vi "4.5 CSM API String to Numeric - Enum.vi"() -> ()   [LabVIEW 2017]
uses:
  <userlib>/_NEVSTOP/Communicable State Machine(CSM)/Communicable State Machine.lvlib
  API-String-Arugments-Support/API String Arguments Support.lvlib
panel:
  out "API String (I32 Channel)":T1(array[cluster])=[{"API String (I32 Channel)"="0", "Channel"=enum."CH1", "Channel"=enum."CH1"}, {"API String (I32 Channel)"="1", "Channel"=enum."CH1", "Channel"=enum."CH2"}, {"API String (I32 Channel)"="2", "Channel"=enum."CH1", "Channel"=enum."CH3"}, {"API String (I32 Channel)"="3", "Channel"=enum."CH1", "Channel"=enum."CH4"}, {"API String (I32 Channel)"="4", "Channel"=enum."CH1", "Channel"=enum."CH5"}, {"API String (I32 Channel)"="5", "Channel"=enum."CH1", "Channel"=enum."CH6"}, {"API String (I32 Channel)"="6", "Channel"=enum."CH1", "Channel"=enum."CH7"}, {"API String (I32 Channel)"="7", "Channel"=enum."CH1", "Channel"=enum."CH8"}, {"API String (I32 Channel)"="8", "Channel"=enum."CH1", "Channel"=enum."CH9"}, {"API String (I32 Channel)"="9", "Channel"=enum."CH1", "Channel"=enum."CH10"}, {"API String (I32 Channel)"="10", "Channel"=enum."CH1", "Channel"=enum."CH11"}, {"API String (I32 Channel)"="11", "Channel"=enum."CH1", "Channel"=enum."CH12"}, {"API String (I32 Channel)"="12", "Channel"=enum."CH1", "Channel"=enum."CH13"}, {"API String (I32 Channel)"="13", "Channel"=enum."CH1", "Channel"=enum."CH14"}, {"API String (I32 Channel)"="14", "Channel"=enum."CH1", "Channel"=enum."CH15"}, {"API String (I32 Channel)"="15", "Channel"=enum."CH1", "Channel"=enum."CH16"}]
  out "API String (Channel)":T2(array[cluster])=[{"API String (Channel)"="CH1", "Channel"=enum."CH1", "Channel"=enum."CH1"}, {"API String (Channel)"="CH2", "Channel"=enum."CH1", "Channel"=enum."CH2"}, {"API String (Channel)"="CH3", "Channel"=enum."CH1", "Channel"=enum."CH3"}, {"API String (Channel)"="CH4", "Channel"=enum."CH1", "Channel"=enum."CH4"}, {"API String (Channel)"="CH5", "Channel"=enum."CH1", "Channel"=enum."CH5"}, {"API String (Channel)"="CH6", "Channel"=enum."CH1", "Channel"=enum."CH6"}, {"API String (Channel)"="CH7", "Channel"=enum."CH1", "Channel"=enum."CH7"}, {"API String (Channel)"="CH8", "Channel"=enum."CH1", "Channel"=enum."CH8"}, {"API String (Channel)"="CH9", "Channel"=enum."CH1", "Channel"=enum."CH9"}, {"API String (Channel)"="CH10", "Channel"=enum."CH1", "Channel"=enum."CH10"}, {"API String (Channel)"="CH11", "Channel"=enum."CH1", "Channel"=enum."CH11"}, {"API String (Channel)"="CH12", "Channel"=enum."CH1", "Channel"=enum."CH12"}, {"API String (Channel)"="CH13", "Channel"=enum."CH1", "Channel"=enum."CH13"}, {"API String (Channel)"="CH14", "Channel"=enum."CH1", "Channel"=enum."CH14"}, {"API String (Channel)"="CH15", "Channel"=enum."CH1", "Channel"=enum."CH15"}, {"API String (Channel)"="CH16", "Channel"=enum."CH1", "Channel"=enum."CH16"}]
  out "API String (I32 Voltage)":T3(array[cluster])=[{"API String (I32 Voltage)"="0", "Enum (Vertical)"=enum."2mV", "Retrieved Vertical"=enum."1mV"}, {"API String (I32 Voltage)"="1", "Enum (Vertical)"=enum."2mV", "Retrieved Vertical"=enum."2mV"}, {"API String (I32 Voltage)"="2", "Enum (Vertical)"=enum."2mV", "Retrieved Vertical"=enum."5mV"}, {"API String (I32 Voltage)"="3", "Enum (Vertical)"=enum."2mV", "Retrieved Vertical"=enum."10mV"}, {"API String (I32 Voltage)"="4", "Enum (Vertical)"=enum."2mV", "Retrieved Vertical"=enum."20mV"}, {"API String (I32 Voltage)"="5", "Enum (Vertical)"=enum."2mV", "Retrieved Vertical"=enum."50mV"}, {"API String (I32 Voltage)"="6", "Enum (Vertical)"=enum."2mV", "Retrieved Vertical"=enum."100mV"}, {"API String (I32 Voltage)"="7", "Enum (Vertical)"=enum."2mV", "Retrieved Vertical"=enum."200mV"}, {"API String (I32 Voltage)"="8", "Enum (Vertical)"=enum."2mV", "Retrieved Vertical"=enum."500mV"}, {"API String (I32 Voltage)"="9", "Enum (Vertical)"=enum."2mV", "Retrieved Vertical"=enum."1V"}, {"API String (I32 Voltage)"="10", "Enum (Vertical)"=enum."2mV", "Retrieved Vertical"=enum."2V"}, {"API String (I32 Voltage)"="11", "Enum (Vertical)"=enum."2mV", "Retrieved Vertical"=enum."5V"}, {"API String (I32 Voltage)"="12", "Enum (Vertical)"=enum."2mV", "Retrieved Vertical"=enum."10V"}, {"API String (I32 Voltage)"="13", "Enum (Vertical)"=enum."2mV", "Retrieved Vertical"=enum."20V"}, {"API String (I32 Voltage)"="14", "Enum (Vertical)"=enum."2mV", "Retrieved Vertical"=enum."50V"}, {"API String (I32 Voltage)"="15", "Enum (Vertical)"=enum."2mV", "Retrieved Vertical"=enum."100V"}, {"API String (I32 Voltage)"="16", "Enum (Vertical)"=enum."2mV", "Retrieved Vertical"=enum."200V"}, {"API String (I32 Voltage)"="17", "Enum (Vertical)"=enum."2mV", "Retrieved Vertical"=enum."500V"}, {"API String (I32 Voltage)"="18", "Enum (Vertical)"=enum."2mV", "Retrieved Vertical"=enum."1kV"}, {"API String (I32 Voltage)"="19", "Enum (Vertical)"=enum."2mV", "Retrieved Vertical"=enum."2kV"}, {"API String (I32 Voltage)"="20", "Enum (Vertical)"=enum."2mV", "Retrieved Vertical"=enum."5kV"}, {"API String (I32 Voltage)"="21", "Enum (Vertical)"=enum."2mV", "Retrieved Vertical"=enum."10kV"}, {"API String (I32 Voltage)"="22", "Enum (Vertical)"=enum."2mV", "Retrieved Vertical"=enum."20kV"}]
  out "API String (SI Voltage)":T4(array[cluster])=[{"API String (SI Voltage)"="1mV", "Enum (Vertical)"=enum."2mV", "Retrieved Vertical"=enum."1mV"}, {"API String (SI Voltage)"="2mV", "Enum (Vertical)"=enum."2mV", "Retrieved Vertical"=enum."2mV"}, {"API String (SI Voltage)"="5mV", "Enum (Vertical)"=enum."2mV", "Retrieved Vertical"=enum."5mV"}, {"API String (SI Voltage)"="10mV", "Enum (Vertical)"=enum."2mV", "Retrieved Vertical"=enum."10mV"}, {"API String (SI Voltage)"="20mV", "Enum (Vertical)"=enum."2mV", "Retrieved Vertical"=enum."20mV"}, {"API String (SI Voltage)"="50mV", "Enum (Vertical)"=enum."2mV", "Retrieved Vertical"=enum."50mV"}, {"API String (SI Voltage)"="100mV", "Enum (Vertical)"=enum."2mV", "Retrieved Vertical"=enum."100mV"}, {"API String (SI Voltage)"="200mV", "Enum (Vertical)"=enum."2mV", "Retrieved Vertical"=enum."200mV"}, {"API String (SI Voltage)"="500mV", "Enum (Vertical)"=enum."2mV", "Retrieved Vertical"=enum."500mV"}, {"API String (SI Voltage)"="1V", "Enum (Vertical)"=enum."2mV", "Retrieved Vertical"=enum."1V"}, {"API String (SI Voltage)"="2V", "Enum (Vertical)"=enum."2mV", "Retrieved Vertical"=enum."2V"}, {"API String (SI Voltage)"="5V", "Enum (Vertical)"=enum."2mV", "Retrieved Vertical"=enum."5V"}, {"API String (SI Voltage)"="10V", "Enum (Vertical)"=enum."2mV", "Retrieved Vertical"=enum."10V"}, {"API String (SI Voltage)"="20V", "Enum (Vertical)"=enum."2mV", "Retrieved Vertical"=enum."20V"}, {"API String (SI Voltage)"="50V", "Enum (Vertical)"=enum."2mV", "Retrieved Vertical"=enum."50V"}, {"API String (SI Voltage)"="100V", "Enum (Vertical)"=enum."2mV", "Retrieved Vertical"=enum."100V"}, {"API String (SI Voltage)"="200V", "Enum (Vertical)"=enum."2mV", "Retrieved Vertical"=enum."200V"}, {"API String (SI Voltage)"="500V", "Enum (Vertical)"=enum."2mV", "Retrieved Vertical"=enum."500V"}, {"API String (SI Voltage)"="1kV", "Enum (Vertical)"=enum."2mV", "Retrieved Vertical"=enum."1kV"}, {"API String (SI Voltage)"="2kV", "Enum (Vertical)"=enum."2mV", "Retrieved Vertical"=enum."2kV"}, {"API String (SI Voltage)"="5kV", "Enum (Vertical)"=enum."2mV", "Retrieved Vertical"=enum."5kV"}, {"API String (SI Voltage)"="10kV", "Enum (Vertical)"=enum."2mV", "Retrieved Vertical"=enum."10kV"}, {"API String (SI Voltage)"="20kV", "Enum (Vertical)"=enum."2mV", "Retrieved Vertical"=enum."20kV"}]
  out "API String (I32 Time)":T5(array[cluster])=[{"API String (I32)"="0", "Enum (Time/Division)"=enum."1us", "Retrieved Enum"=enum."100ns"}, {"API String (I32)"="1", "Enum (Time/Division)"=enum."1us", "Retrieved Enum"=enum."200ns"}, {"API String (I32)"="2", "Enum (Time/Division)"=enum."1us", "Retrieved Enum"=enum."500ns"}, {"API String (I32)"="3", "Enum (Time/Division)"=enum."1us", "Retrieved Enum"=enum."1us"}, {"API String (I32)"="4", "Enum (Time/Division)"=enum."1us", "Retrieved Enum"=enum."2us"}, {"API String (I32)"="5", "Enum (Time/Division)"=enum."1us", "Retrieved Enum"=enum."5us"}, {"API String (I32)"="6", "Enum (Time/Division)"=enum."1us", "Retrieved Enum"=enum."10us"}, {"API String (I32)"="7", "Enum (Time/Division)"=enum."1us", "Retrieved Enum"=enum."20us"}, {"API String (I32)"="8", "Enum (Time/Division)"=enum."1us", "Retrieved Enum"=enum."50us"}, {"API String (I32)"="9", "Enum (Time/Division)"=enum."1us", "Retrieved Enum"=enum."100us"}, {"API String (I32)"="10", "Enum (Time/Division)"=enum."1us", "Retrieved Enum"=enum."200us"}, {"API String (I32)"="11", "Enum (Time/Division)"=enum."1us", "Retrieved Enum"=enum."500us"}, {"API String (I32)"="12", "Enum (Time/Division)"=enum."1us", "Retrieved Enum"=enum."1ms"}, {"API String (I32)"="13", "Enum (Time/Division)"=enum."1us", "Retrieved Enum"=enum."2ms"}, {"API String (I32)"="14", "Enum (Time/Division)"=enum."1us", "Retrieved Enum"=enum."5ms"}, {"API String (I32)"="15", "Enum (Time/Division)"=enum."1us", "Retrieved Enum"=enum."10ms"}, {"API String (I32)"="16", "Enum (Time/Division)"=enum."1us", "Retrieved Enum"=enum."20ms"}, {"API String (I32)"="17", "Enum (Time/Division)"=enum."1us", "Retrieved Enum"=enum."50ms"}, {"API String (I32)"="18", "Enum (Time/Division)"=enum."1us", "Retrieved Enum"=enum."100ms"}, {"API String (I32)"="19", "Enum (Time/Division)"=enum."1us", "Retrieved Enum"=enum."200ms"}, {"API String (I32)"="20", "Enum (Time/Division)"=enum."1us", "Retrieved Enum"=enum."500ms"}, {"API String (I32)"="21", "Enum (Time/Division)"=enum."1us", "Retrieved Enum"=enum."1s"}, {"API String (I32)"="22", "Enum (Time/Division)"=enum."1us", "Retrieved Enum"=enum."2s"}, {"API String (I32)"="23", "Enum (Time/Division)"=enum."1us", "Retrieved Enum"=enum."3s"}, {"API String (I32)"="24", "Enum (Time/Division)"=enum."1us", "Retrieved Enum"=enum."4s"}, {"API String (I32)"="25", "Enum (Time/Division)"=enum."1us", "Retrieved Enum"=enum."5s"}, {"API String (I32)"="26", "Enum (Time/Division)"=enum."1us", "Retrieved Enum"=enum."6s"}, {"API String (I32)"="27", "Enum (Time/Division)"=enum."1us", "Retrieved Enum"=enum."8s"}, {"API String (I32)"="28", "Enum (Time/Division)"=enum."1us", "Retrieved Enum"=enum."10s"}, {"API String (I32)"="29", "Enum (Time/Division)"=enum."1us", "Retrieved Enum"=enum."20s"}, {"API String (I32)"="30", "Enum (Time/Division)"=enum."1us", "Retrieved Enum"=enum."30s"}, {"API String (I32)"="31", "Enum (Time/Division)"=enum."1us", "Retrieved Enum"=enum."1min"}, {"API String (I32)"="32", "Enum (Time/Division)"=enum."1us", "Retrieved Enum"=enum."2min"}, {"API String (I32)"="33", "Enum (Time/Division)"=enum."1us", "Retrieved Enum"=enum."3min"}, {"API String (I32)"="34", "Enum (Time/Division)"=enum."1us", "Retrieved Enum"=enum."4min"}, {"API String (I32)"="35", "Enum (Time/Division)"=enum."1us", "Retrieved Enum"=enum."5min"}, {"API String (I32)"="36", "Enum (Time/Division)"=enum."1us", "Retrieved Enum"=enum."6min"}, {"API String (I32)"="37", "Enum (Time/Division)"=enum."1us", "Retrieved Enum"=enum."7min"}, {"API String (I32)"="38", "Enum (Time/Division)"=enum."1us", "Retrieved Enum"=enum."8min"}, {"API String (I32)"="39", "Enum (Time/Division)"=enum."1us", "Retrieved Enum"=enum."9min"}, {"API String (I32)"="40", "Enum (Time/Division)"=enum."1us", "Retrieved Enum"=enum."10min"}, {"API String (I32)"="41", "Enum (Time/Division)"=enum."1us", "Retrieved Enum"=enum."12min"}, {"API String (I32)"="42", "Enum (Time/Division)"=enum."1us", "Retrieved Enum"=enum."15min"}, {"API String (I32)"="43", "Enum (Time/Division)"=enum."1us", "Retrieved Enum"=enum."30min"}, {"API String (I32)"="44", "Enum (Time/Division)"=enum."1us", "Retrieved Enum"=enum."1hour"}, {"API String (I32)"="45", "Enum (Time/Division)"=enum."1us", "Retrieved Enum"=enum."2hour"}, {"API String (I32)"="46", "Enum (Time/Division)"=enum."1us", "Retrieved Enum"=enum."3hour"}, {"API String (I32)"="47", "Enum (Time/Division)"=enum."1us", "Retrieved Enum"=enum."4hour"}, {"API String (I32)"="48", "Enum (Time/Division)"=enum."1us", "Retrieved Enum"=enum."5hour"}, {"API String (I32)"="49", "Enum (Time/Division)"=enum."1us", "Retrieved Enum"=enum."6hour"}, {"API String (I32)"="50", "Enum (Time/Division)"=enum."1us", "Retrieved Enum"=enum."7hour"}, {"API String (I32)"="51", "Enum (Time/Division)"=enum."1us", "Retrieved Enum"=enum."8hour"}, {"API String (I32)"="52", "Enum (Time/Division)"=enum."1us", "Retrieved Enum"=enum."9hour"}, {"API String (I32)"="53", "Enum (Time/Division)"=enum."1us", "Retrieved Enum"=enum."10hour"}, {"API String (I32)"="54", "Enum (Time/Division)"=enum."1us", "Retrieved Enum"=enum."12hour"}, {"API String (I32)"="55", "Enum (Time/Division)"=enum."1us", "Retrieved Enum"=enum."1day"}, {"API String (I32)"="56", "Enum (Time/Division)"=enum."1us", "Retrieved Enum"=enum."2day"}, {"API String (I32)"="57", "Enum (Time/Division)"=enum."1us", "Retrieved Enum"=enum."3day"}]
  out "API String (SI Time)":T6(array[cluster])=[{"API String (SI Format)"="100ns", "Enum (Time/Division)"=enum."1us", "Retrieved Enum"=enum."100ns"}, {"API String (SI Format)"="200ns", "Enum (Time/Division)"=enum."1us", "Retrieved Enum"=enum."200ns"}, {"API String (SI Format)"="500ns", "Enum (Time/Division)"=enum."1us", "Retrieved Enum"=enum."500ns"}, {"API String (SI Format)"="1us", "Enum (Time/Division)"=enum."1us", "Retrieved Enum"=enum."1us"}, {"API String (SI Format)"="2us", "Enum (Time/Division)"=enum."1us", "Retrieved Enum"=enum."2us"}, {"API String (SI Format)"="5us", "Enum (Time/Division)"=enum."1us", "Retrieved Enum"=enum."5us"}, {"API String (SI Format)"="10us", "Enum (Time/Division)"=enum."1us", "Retrieved Enum"=enum."10us"}, {"API String (SI Format)"="20us", "Enum (Time/Division)"=enum."1us", "Retrieved Enum"=enum."20us"}, {"API String (SI Format)"="50us", "Enum (Time/Division)"=enum."1us", "Retrieved Enum"=enum."50us"}, {"API String (SI Format)"="100us", "Enum (Time/Division)"=enum."1us", "Retrieved Enum"=enum."100us"}, {"API String (SI Format)"="200us", "Enum (Time/Division)"=enum."1us", "Retrieved Enum"=enum."200us"}, {"API String (SI Format)"="500us", "Enum (Time/Division)"=enum."1us", "Retrieved Enum"=enum."500us"}, {"API String (SI Format)"="1ms", "Enum (Time/Division)"=enum."1us", "Retrieved Enum"=enum."1ms"}, {"API String (SI Format)"="2ms", "Enum (Time/Division)"=enum."1us", "Retrieved Enum"=enum."2ms"}, {"API String (SI Format)"="5ms", "Enum (Time/Division)"=enum."1us", "Retrieved Enum"=enum."5ms"}, {"API String (SI Format)"="10ms", "Enum (Time/Division)"=enum."1us", "Retrieved Enum"=enum."10ms"}, {"API String (SI Format)"="20ms", "Enum (Time/Division)"=enum."1us", "Retrieved Enum"=enum."20ms"}, {"API String (SI Format)"="50ms", "Enum (Time/Division)"=enum."1us", "Retrieved Enum"=enum."50ms"}, {"API String (SI Format)"="100ms", "Enum (Time/Division)"=enum."1us", "Retrieved Enum"=enum."100ms"}, {"API String (SI Format)"="200ms", "Enum (Time/Division)"=enum."1us", "Retrieved Enum"=enum."200ms"}, {"API String (SI Format)"="500ms", "Enum (Time/Division)"=enum."1us", "Retrieved Enum"=enum."500ms"}, {"API String (SI Format)"="1s", "Enum (Time/Division)"=enum."1us", "Retrieved Enum"=enum."1s"}, {"API String (SI Format)"="2s", "Enum (Time/Division)"=enum."1us", "Retrieved Enum"=enum."2s"}, {"API String (SI Format)"="3s", "Enum (Time/Division)"=enum."1us", "Retrieved Enum"=enum."3s"}, {"API String (SI Format)"="4s", "Enum (Time/Division)"=enum."1us", "Retrieved Enum"=enum."4s"}, {"API String (SI Format)"="5s", "Enum (Time/Division)"=enum."1us", "Retrieved Enum"=enum."5s"}, {"API String (SI Format)"="6s", "Enum (Time/Division)"=enum."1us", "Retrieved Enum"=enum."6s"}, {"API String (SI Format)"="8s", "Enum (Time/Division)"=enum."1us", "Retrieved Enum"=enum."8s"}, {"API String (SI Format)"="10s", "Enum (Time/Division)"=enum."1us", "Retrieved Enum"=enum."10s"}, {"API String (SI Format)"="20s", "Enum (Time/Division)"=enum."1us", "Retrieved Enum"=enum."20s"}, {"API String (SI Format)"="30s", "Enum (Time/Division)"=enum."1us", "Retrieved Enum"=enum."30s"}, {"API String (SI Format)"="1min", "Enum (Time/Division)"=enum."1us", "Retrieved Enum"=enum."1min"}, {"API String (SI Format)"="2min", "Enum (Time/Division)"=enum."1us", "Retrieved Enum"=enum."2min"}, {"API String (SI Format)"="3min", "Enum (Time/Division)"=enum."1us", "Retrieved Enum"=enum."3min"}, {"API String (SI Format)"="4min", "Enum (Time/Division)"=enum."1us", "Retrieved Enum"=enum."4min"}, {"API String (SI Format)"="5min", "Enum (Time/Division)"=enum."1us", "Retrieved Enum"=enum."5min"}, {"API String (SI Format)"="6min", "Enum (Time/Division)"=enum."1us", "Retrieved Enum"=enum."6min"}, {"API String (SI Format)"="7min", "Enum (Time/Division)"=enum."1us", "Retrieved Enum"=enum."7min"}, {"API String (SI Format)"="8min", "Enum (Time/Division)"=enum."1us", "Retrieved Enum"=enum."8min"}, {"API String (SI Format)"="9min", "Enum (Time/Division)"=enum."1us", "Retrieved Enum"=enum."9min"}, {"API String (SI Format)"="10min", "Enum (Time/Division)"=enum."1us", "Retrieved Enum"=enum."10min"}, {"API String (SI Format)"="12min", "Enum (Time/Division)"=enum."1us", "Retrieved Enum"=enum."12min"}, {"API String (SI Format)"="15min", "Enum (Time/Division)"=enum."1us", "Retrieved Enum"=enum."15min"}, {"API String (SI Format)"="30min", "Enum (Time/Division)"=enum."1us", "Retrieved Enum"=enum."30min"}, {"API String (SI Format)"="1hour", "Enum (Time/Division)"=enum."1us", "Retrieved Enum"=enum."1hour"}, {"API String (SI Format)"="2hour", "Enum (Time/Division)"=enum."1us", "Retrieved Enum"=enum."2hour"}, {"API String (SI Format)"="3hour", "Enum (Time/Division)"=enum."1us", "Retrieved Enum"=enum."3hour"}, {"API String (SI Format)"="4hour", "Enum (Time/Division)"=enum."1us", "Retrieved Enum"=enum."4hour"}, {"API String (SI Format)"="5hour", "Enum (Time/Division)"=enum."1us", "Retrieved Enum"=enum."5hour"}, {"API String (SI Format)"="6hour", "Enum (Time/Division)"=enum."1us", "Retrieved Enum"=enum."6hour"}, {"API String (SI Format)"="7hour", "Enum (Time/Division)"=enum."1us", "Retrieved Enum"=enum."7hour"}, {"API String (SI Format)"="8hour", "Enum (Time/Division)"=enum."1us", "Retrieved Enum"=enum."8hour"}, {"API String (SI Format)"="9hour", "Enum (Time/Division)"=enum."1us", "Retrieved Enum"=enum."9hour"}, {"API String (SI Format)"="10hour", "Enum (Time/Division)"=enum."1us", "Retrieved Enum"=enum."10hour"}, {"API String (SI Format)"="12hour", "Enum (Time/Division)"=enum."1us", "Retrieved Enum"=enum."12hour"}, {"API String (SI Format)"="1day", "Enum (Time/Division)"=enum."1us", "Retrieved Enum"=enum."1day"}, {"API String (SI Format)"="2day", "Enum (Time/Division)"=enum."1us", "Retrieved Enum"=enum."2day"}, {"API String (SI Format)"="3day", "Enum (Time/Division)"=enum."1us", "Retrieved Enum"=enum."3day"}]
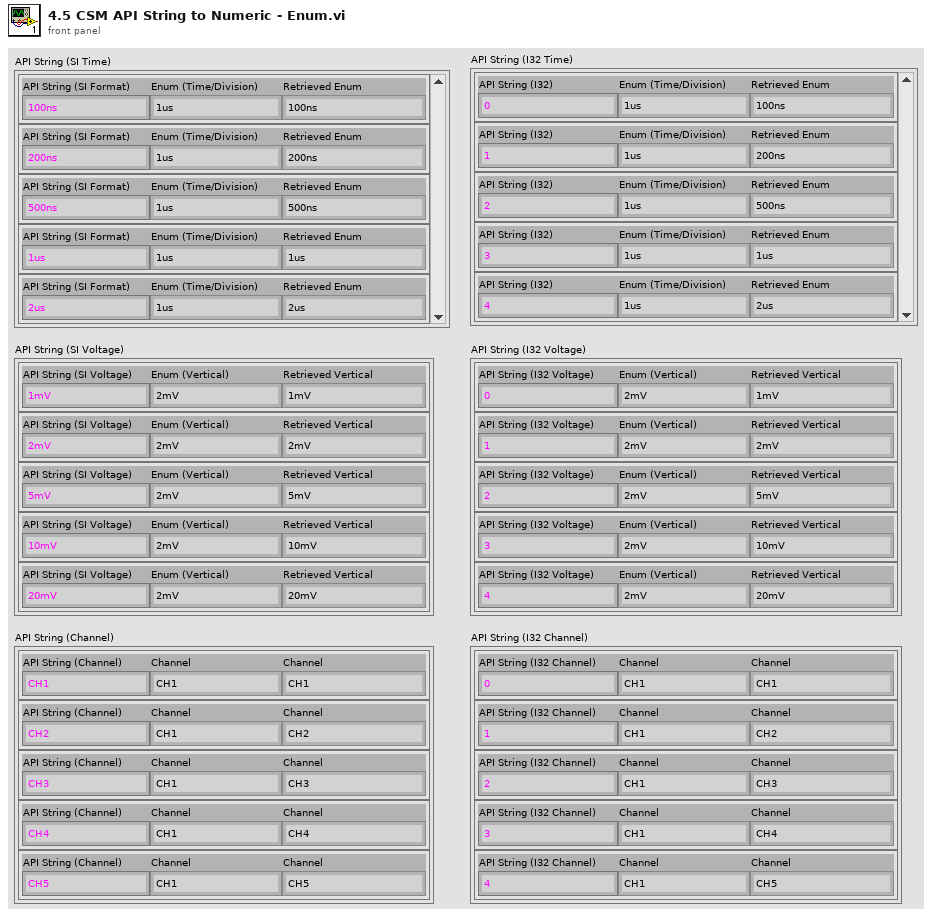
[diagram p1: front panel]
types:
  T1 = cluster{"API String (I32 Channel)":string, "Channel":enum16{"CH1", "CH2", "CH3", "CH4", "CH5", "CH6", "CH7", "CH8", "CH9", "CH10", "CH11", "CH12", "CH13", "CH14", "CH15", "CH16"}, "Channel":enum16{"CH1", "CH2", "CH3", "CH4", "CH5", "CH6", "CH7", "CH8", "CH9", "CH10", "CH11", "CH12", "CH13", "CH14", "CH15", "CH16"}}[]
  T2 = cluster{"API String (Channel)":string, "Channel":enum16{"CH1", "CH2", "CH3", "CH4", "CH5", "CH6", "CH7", "CH8", "CH9", "CH10", "CH11", "CH12", "CH13", "CH14", "CH15", "CH16"}, "Channel":enum16{"CH1", "CH2", "CH3", "CH4", "CH5", "CH6", "CH7", "CH8", "CH9", "CH10", "CH11", "CH12", "CH13", "CH14", "CH15", "CH16"}}[]
  T3 = cluster{"API String (I32 Voltage)":string, "Enum (Vertical)":enum16{"1mV", "2mV", "5mV", "10mV", "20mV", "50mV", "100mV", "200mV", "500mV", "1V", "2V", "5V", "10V", "20V", "50V", "100V", "200V", "500V", "1kV", "2kV", "5kV", "10kV", "20kV"}, "Retrieved Vertical":enum16{"1mV", "2mV", "5mV", "10mV", "20mV", "50mV", "100mV", "200mV", "500mV", "1V", "2V", "5V", "10V", "20V", "50V", "100V", "200V", "500V", "1kV", "2kV", "5kV", "10kV", "20kV"}}[]
  T4 = cluster{"API String (SI Voltage)":string, "Enum (Vertical)":enum16{"1mV", "2mV", "5mV", "10mV", "20mV", "50mV", "100mV", "200mV", "500mV", "1V", "2V", "5V", "10V", "20V", "50V", "100V", "200V", "500V", "1kV", "2kV", "5kV", "10kV", "20kV"}, "Retrieved Vertical":enum16{"1mV", "2mV", "5mV", "10mV", "20mV", "50mV", "100mV", "200mV", "500mV", "1V", "2V", "5V", "10V", "20V", "50V", "100V", "200V", "500V", "1kV", "2kV", "5kV", "10kV", "20kV"}}[]
  T5 = cluster{"API String (I32)":string, "Enum (Time/Division)":enum16{"100ns", "200ns", "500ns", "1us", "2us", "5us", "10us", "20us", "50us", "100us", "200us", "500us", "1ms", "2ms", "5ms", "10ms", "20ms", "50ms", "100ms", "200ms", "500ms", "1s", "2s", "3s", "4s", "5s", "6s", "8s", "10s", "20s", "30s", "1min", "2min", "3min", "4min", "5min", "6min", "7min", "8min", "9min", "10min", "12min", "15min", "30min", "1hour", "2hour", "3hour", "4hour", "5hour", "6hour", "7hour", "8hour", "9hour", "10hour", "12hour", "1day", "2day", "3day"}, "Retrieved Enum":enum16{"100ns", "200ns", "500ns", "1us", "2us", "5us", "10us", "20us", "50us", "100us", "200us", "500us", "1ms", "2ms", "5ms", "10ms", "20ms", "50ms", "100ms", "200ms", "500ms", "1s", "2s", "3s", "4s", "5s", "6s", "8s", "10s", "20s", "30s", "1min", "2min", "3min", "4min", "5min", "6min", "7min", "8min", "9min", "10min", "12min", "15min", "30min", "1hour", "2hour", "3hour", "4hour", "5hour", "6hour", "7hour", "8hour", "9hour", "10hour", "12hour", "1day", "2day", "3day"}}[]
  T6 = cluster{"API String (SI Format)":string, "Enum (Time/Division)":enum16{"100ns", "200ns", "500ns", "1us", "2us", "5us", "10us", "20us", "50us", "100us", "200us", "500us", "1ms", "2ms", "5ms", "10ms", "20ms", "50ms", "100ms", "200ms", "500ms", "1s", "2s", "3s", "4s", "5s", "6s", "8s", "10s", "20s", "30s", "1min", "2min", "3min", "4min", "5min", "6min", "7min", "8min", "9min", "10min", "12min", "15min", "30min", "1hour", "2hour", "3hour", "4hour", "5hour", "6hour", "7hour", "8hour", "9hour", "10hour", "12hour", "1day", "2day", "3day"}, "Retrieved Enum":enum16{"100ns", "200ns", "500ns", "1us", "2us", "5us", "10us", "20us", "50us", "100us", "200us", "500us", "1ms", "2ms", "5ms", "10ms", "20ms", "50ms", "100ms", "200ms", "500ms", "1s", "2s", "3s", "4s", "5s", "6s", "8s", "10s", "20s", "30s", "1min", "2min", "3min", "4min", "5min", "6min", "7min", "8min", "9min", "10min", "12min", "15min", "30min", "1hour", "2hour", "3hour", "4hour", "5hour", "6hour", "7hour", "8hour", "9hour", "10hour", "12hour", "1day", "2day", "3day"}}[]
  T7 = enum16{"CH1", "CH2", "CH3", "CH4", "CH5", "CH6", "CH7", "CH8", "CH9", "CH10", "CH11", "CH12", "CH13", "CH14", "CH15", "CH16"}
  T8 = enum16{"100ns", "200ns", "500ns", "1us", "2us", "5us", "10us", "20us", "50us", "100us", "200us", "500us", "1ms", "2ms", "5ms", "10ms", "20ms", "50ms", "100ms", "200ms", "500ms", "1s", "2s", "3s", "4s", "5s", "6s", "8s", "10s", "20s", "30s", "1min", "2min", "3min", "4min", "5min", "6min", "7min", "8min", "9min", "10min", "12min", "15min", "30min", "1hour", "2hour", "3hour", "4hour", "5hour", "6hour", "7hour", "8hour", "9hour", "10hour", "12hour", "1day", "2day", "3day"}
  T9 = enum16{"1mV", "2mV", "5mV", "10mV", "20mV", "50mV", "100mV", "200mV", "500mV", "1V", "2V", "5V", "10V", "20V", "50V", "100V", "200V", "500V", "1kV", "2kV", "5kV", "10kV", "20kV"}
  T10 = cluster{"string":string, "Time/Division (12: 1ms)":enum16{"100ns", "200ns", "500ns", "1us", "2us", "5us", "10us", "20us", "50us", "100us", "200us", "500us", "1ms", "2ms", "5ms", "10ms", "20ms", "50ms", "100ms", "200ms", "500ms", "1s", "2s", "3s", "4s", "5s", "6s", "8s", "10s", "20s", "30s", "1min", "2min", "3min", "4min", "5min", "6min", "7min", "8min", "9min", "10min", "12min", "15min", "30min", "1hour", "2hour", "3hour", "4hour", "5hour", "6hour", "7hour", "8hour", "9hour", "10hour", "12hour", "1day", "2day", "3day"}, "Time/Division (12: 1ms)":enum16{"100ns", "200ns", "500ns", "1us", "2us", "5us", "10us", "20us", "50us", "100us", "200us", "500us", "1ms", "2ms", "5ms", "10ms", "20ms", "50ms", "100ms", "200ms", "500ms", "1s", "2s", "3s", "4s", "5s", "6s", "8s", "10s", "20s", "30s", "1min", "2min", "3min", "4min", "5min", "6min", "7min", "8min", "9min", "10min", "12min", "15min", "30min", "1hour", "2hour", "3hour", "4hour", "5hour", "6hour", "7hour", "8hour", "9hour", "10hour", "12hour", "1day", "2day", "3day"}}
  T11 = cluster{string, "Time/Division (12: 1ms)":enum16{"100ns", "200ns", "500ns", "1us", "2us", "5us", "10us", "20us", "50us", "100us", "200us", "500us", "1ms", "2ms", "5ms", "10ms", "20ms", "50ms", "100ms", "200ms", "500ms", "1s", "2s", "3s", "4s", "5s", "6s", "8s", "10s", "20s", "30s", "1min", "2min", "3min", "4min", "5min", "6min", "7min", "8min", "9min", "10min", "12min", "15min", "30min", "1hour", "2hour", "3hour", "4hour", "5hour", "6hour", "7hour", "8hour", "9hour", "10hour", "12hour", "1day", "2day", "3day"}, "Time/Division (12: 1ms)":enum16{"100ns", "200ns", "500ns", "1us", "2us", "5us", "10us", "20us", "50us", "100us", "200us", "500us", "1ms", "2ms", "5ms", "10ms", "20ms", "50ms", "100ms", "200ms", "500ms", "1s", "2s", "3s", "4s", "5s", "6s", "8s", "10s", "20s", "30s", "1min", "2min", "3min", "4min", "5min", "6min", "7min", "8min", "9min", "10min", "12min", "15min", "30min", "1hour", "2hour", "3hour", "4hour", "5hour", "6hour", "7hour", "8hour", "9hour", "10hour", "12hour", "1day", "2day", "3day"}}
  T12 = cluster{"string":string, "Vertical":enum16{"1mV", "2mV", "5mV", "10mV", "20mV", "50mV", "100mV", "200mV", "500mV", "1V", "2V", "5V", "10V", "20V", "50V", "100V", "200V", "500V", "1kV", "2kV", "5kV", "10kV", "20kV"}, "Vertical":enum16{"1mV", "2mV", "5mV", "10mV", "20mV", "50mV", "100mV", "200mV", "500mV", "1V", "2V", "5V", "10V", "20V", "50V", "100V", "200V", "500V", "1kV", "2kV", "5kV", "10kV", "20kV"}}
  T13 = cluster{string, "Vertical":enum16{"1mV", "2mV", "5mV", "10mV", "20mV", "50mV", "100mV", "200mV", "500mV", "1V", "2V", "5V", "10V", "20V", "50V", "100V", "200V", "500V", "1kV", "2kV", "5kV", "10kV", "20kV"}, "Vertical":enum16{"1mV", "2mV", "5mV", "10mV", "20mV", "50mV", "100mV", "200mV", "500mV", "1V", "2V", "5V", "10V", "20V", "50V", "100V", "200V", "500V", "1kV", "2kV", "5kV", "10kV", "20kV"}}
  T14 = cluster{"string":string, "Channel":enum16{"CH1", "CH2", "CH3", "CH4", "CH5", "CH6", "CH7", "CH8", "CH9", "CH10", "CH11", "CH12", "CH13", "CH14", "CH15", "CH16"}, "Channel":enum16{"CH1", "CH2", "CH3", "CH4", "CH5", "CH6", "CH7", "CH8", "CH9", "CH10", "CH11", "CH12", "CH13", "CH14", "CH15", "CH16"}}
  T15 = cluster{string, "Channel":enum16{"CH1", "CH2", "CH3", "CH4", "CH5", "CH6", "CH7", "CH8", "CH9", "CH10", "CH11", "CH12", "CH13", "CH14", "CH15", "CH16"}, "Channel":enum16{"CH1", "CH2", "CH3", "CH4", "CH5", "CH6", "CH7", "CH8", "CH9", "CH10", "CH11", "CH12", "CH13", "CH14", "CH15", "CH16"}}
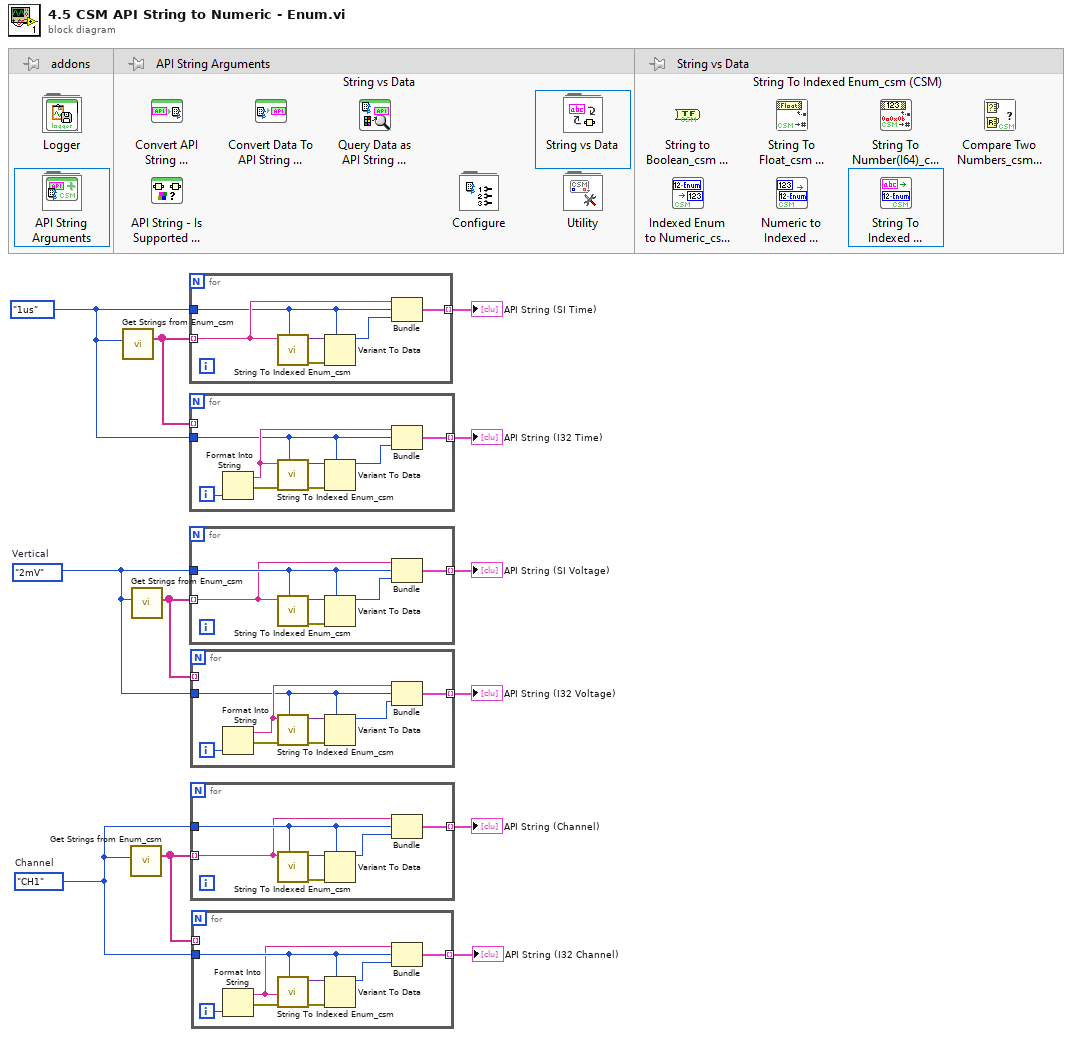
[diagram p0: block diagram]
diagram:
  w7 = T7."CH1"  # Channel
  w12 = T8."1us" ("Time/Division (12: 1ms)")
  w9 = T9."2mV"  # Vertical
  n1 = call <userlib>:"Get Strings from Enum_csm.vi"("Enum"=w12) -> ("Enum Strings"=w11:string[])  [unwired: 7 in, 3 out]
  n2 = call <userlib>:"Get Strings from Enum_csm.vi"("Enum"=w7) -> ("Enum Strings"=w8:string[])  [unwired: 7 in, 3 out]
  n3 = call <userlib>:"Get Strings from Enum_csm.vi"("Enum"=w9) -> ("Enum Strings"=w10:string[])  [unwired: 7 in, 3 out]
  n4 = for {
    tunnel: w12 -> [w15]
    tunnel: w11 -> [w16] mode=indexing
    tunnel: [w13] -> w6 mode=indexing
    n5 = call "String To Indexed Enum_csm.vi"("Variant"=w15, "String"=w16) -> ("error out"=w17:errorcluster, "Enum"=w18:variant)  [unwired: 8 in]
    n6 = Variant To Data(error in=w17, type=w15, Variant=w18) -> (data=w14:T8)  [unwired: 1 out]
    n7 = Bundle("string"=w16, "Time/Division (12: 1ms)"=w15, "Time/Division (12: 1ms)"=w14) -> (w13:T10)  [unwired: 1 in]
  }
  "API String (SI Time)" <- w6
  n8 = for {
    tunnel: w12 -> [w21]
    tunnel: w11 -> [_] mode=indexing
    tunnel: [w19] -> w5 mode=indexing
    i -> [w23]
    n9 = Format Into String(w23) -> (resulting string=w22:string, error out=w24:errorcluster)  [unwired: 3 in]
    n10 = call "String To Indexed Enum_csm.vi"("Variant"=w21, "error in (no error)"=w24, "String"=w22) -> ("error out"=w25:errorcluster, "Enum"=w26:variant)  [unwired: 7 in]
    n11 = Variant To Data(error in=w25, type=w21, Variant=w26) -> (data=w20:T8)  [unwired: 1 out]
    n12 = Bundle(w22, "Time/Division (12: 1ms)"=w21, "Time/Division (12: 1ms)"=w20) -> (w19:T11)  [unwired: 1 in]
  }
  "API String (I32 Time)" <- w5
  n13 = for {
    tunnel: w9 -> [w30]
    tunnel: w10 -> [w29] mode=indexing
    tunnel: [w27] -> w4 mode=indexing
    n14 = call "String To Indexed Enum_csm.vi"("Variant"=w30, "String"=w29) -> ("error out"=w31:errorcluster, "Enum"=w32:variant)  [unwired: 8 in]
    n15 = Variant To Data(error in=w31, type=w30, Variant=w32) -> (data=w28:T9)  [unwired: 1 out]
    n16 = Bundle("string"=w29, "Vertical"=w30, "Vertical"=w28) -> (w27:T12)  [unwired: 1 in]
  }
  "API String (SI Voltage)" <- w4
  n17 = for {
    tunnel: w9 -> [w35]
    tunnel: w10 -> [_] mode=indexing
    tunnel: [w33] -> w3 mode=indexing
    i -> [w38]
    n18 = Format Into String(w38) -> (resulting string=w36:string, error out=w37:errorcluster)  [unwired: 3 in]
    n19 = call "String To Indexed Enum_csm.vi"("Variant"=w35, "error in (no error)"=w37, "String"=w36) -> ("error out"=w39:errorcluster, "Enum"=w40:variant)  [unwired: 7 in]
    n20 = Variant To Data(error in=w39, type=w35, Variant=w40) -> (data=w34:T9)  [unwired: 1 out]
    n21 = Bundle(w36, "Vertical"=w35, "Vertical"=w34) -> (w33:T13)  [unwired: 1 in]
  }
  "API String (I32 Voltage)" <- w3
  n22 = for {
    tunnel: w7 -> [w44]
    tunnel: w8 -> [w43] mode=indexing
    tunnel: [w41] -> w2 mode=indexing
    n23 = call "String To Indexed Enum_csm.vi"("Variant"=w44, "String"=w43) -> ("error out"=w45:errorcluster, "Enum"=w46:variant)  [unwired: 8 in]
    n24 = Variant To Data(error in=w45, type=w44, Variant=w46) -> (data=w42:T7)  [unwired: 1 out]
    n25 = Bundle("string"=w43, "Channel"=w44, "Channel"=w42) -> (w41:T14)  [unwired: 1 in]
  }
  "API String (Channel)" <- w2
  n26 = for {
    tunnel: w7 -> [w50]
    tunnel: w8 -> [_] mode=indexing
    tunnel: [w47] -> w1 mode=indexing
    i -> [w51]
    n27 = Format Into String(w51) -> (resulting string=w49:string, error out=w52:errorcluster)  [unwired: 3 in]
    n28 = call "String To Indexed Enum_csm.vi"("Variant"=w50, "error in (no error)"=w52, "String"=w49) -> ("error out"=w53:errorcluster, "Enum"=w54:variant)  [unwired: 7 in]
    n29 = Variant To Data(error in=w53, type=w50, Variant=w54) -> (data=w48:T7)  [unwired: 1 out]
    n30 = Bundle(w49, "Channel"=w50, "Channel"=w48) -> (w47:T15)  [unwired: 1 in]
  }
  "API String (I32 Channel)" <- w1
